vi "HasControlsOnConnectorPane.vi"(8 "error in (no error)":errorcluster, 10 "VI Refnum":refnum<vi>) -> (0 "error out":errorcluster, 2 "Is Connected?":bool)   [LabVIEW 2019, in "LVUnitTestBuilder.lvclass"]
doc: "Returns true if the specified VI has at least one control connected to the connector pane."
uses:
  LVUnitTestBuilder.lvclass
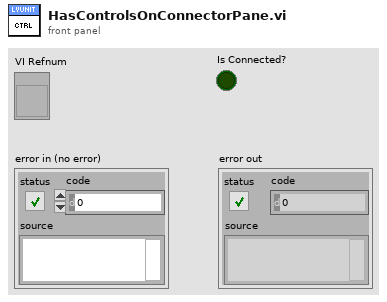
[diagram p1: front panel]
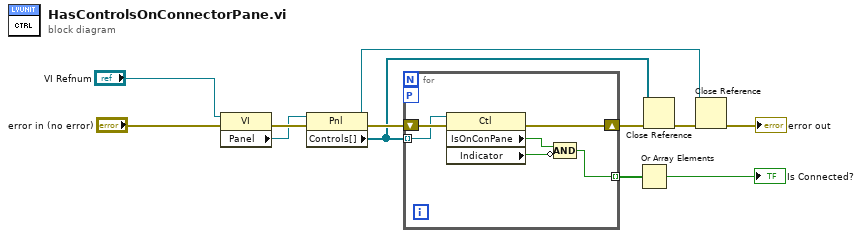
[diagram p0: block diagram]
diagram:
  n1 = property class="VI"(reference="VI Refnum", error in="error in (no error)") -> (error out=w12:errorcluster, "Panel"=w11:refnum<vi>)  [unwired: 1 out]
  n2 = property class="Pnl"(reference=w11, error in=w12) -> (reference out=w9:refnum<vi>, error out=w10:errorcluster, "Controls[]"=w6:refnum<vi>[])
  n3 = for {
    tunnel: w6 -> [w17] mode=indexing
    shift-right: [w16] -> w8
    shift-left: w10 -> [w18]
    tunnel: [w13] -> w4 mode=indexing
    workers-P: _ -> [_]
    n4 = property class="Ctl"(reference=w17, error in=w18) -> (error out=w16:errorcluster, "IsOnConPane"=w14:bool, "Indicator"=w15:bool)  [unwired: 1 out]
    n5 = Compound Arithmetic op=AND(w14, invert w15) -> (w13:bool)
  }
  n6 = Or Array Elements(Boolean array=w4) -> (logical OR=→"Is Connected?":bool)
  n7 = Close Reference(reference=w6, error in (no error)=w8) -> (error out=w7:errorcluster)
  n8 = Close Reference(reference=w9, error in (no error)=w7) -> (error out=→"error out":errorcluster)
